vi "AppendRawData.vi"(8 "error in (no error)":errorcluster, 10 "NewRawData":waveform(dbl)[](array[waveform]), 11 "OldRawData":waveform(dbl)[](array[waveform])) -> (0 "error out":errorcluster, 3 "AppendedData":waveform(dbl)[](array[waveform]))   [LabVIEW 2022 SP3]
uses:
  <vilib>/Waveform/WDTOps.llb/WDT Append Waveforms DBL.vi
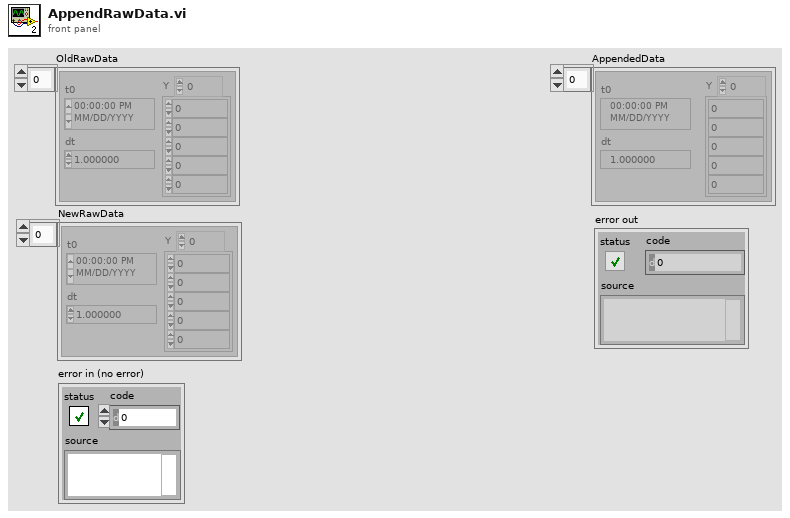
[diagram p1: front panel]
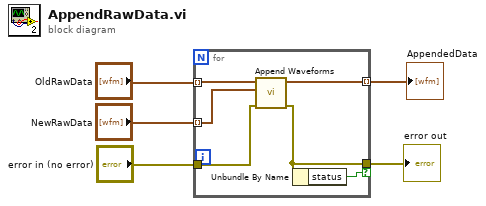
[diagram p0: block diagram]
diagram:
  n1 = for {
    tunnel: "NewRawData" -> [w9] mode=indexing
    tunnel: "OldRawData" -> [w10] mode=indexing
    tunnel: [w11] -> w1 mode=indexing
    tunnel: "error in (no error)" -> [w8]
    tunnel: [w6] -> w2 if=w7
    n2 = call-poly <vilib>:"Append Waveforms.vi"("error in (no error)"=w8, "waveform B"=w9, "waveform A"=w10) -> ("error out"=w6:errorcluster, "waveform out"=w11:waveform(dbl))  [unwired: 7 in]
    n3 = Unbundle By Name(w6) -> ("status"=w7:bool)
  }
  "error out" <- w2
  "AppendedData" <- w1
